vi "Configure Trigger.vi"(0 "VISA resource name":refnum<visa-resource-name>, 1 "Trigger Level (0.0 dBm)":dbl, 5 "Channel (1: Channel A)":u16(ring)=1 items=["Channel A"=1, "Channel B"=2], 7 "Trigger Source (3: Immediate)":u16(ring)=3 items=["Bus", "External", "Hold", "Immediate", "Internal A", "Internal B"], 9 "Trigger Slope (0: Positive)":u16(ring) items=["Positive", "Negative"], 11 "error in (no error)":errorcluster) -> (4 "VISA resource name out":refnum<visa-resource-name>, 15 "error out":errorcluster)   [LabVIEW 2020, in "Template - Power Meter.lvlib"]
doc: "Controls the behavior of the trigger system, including Trigger Source, Trigger Slope, and Trigger Level."
uses:
  <instrlib>/_Template - Power Meter/Template - Power Meter.lvlib
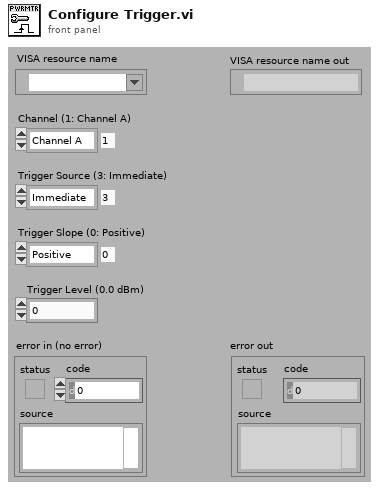
[diagram p1: front panel]
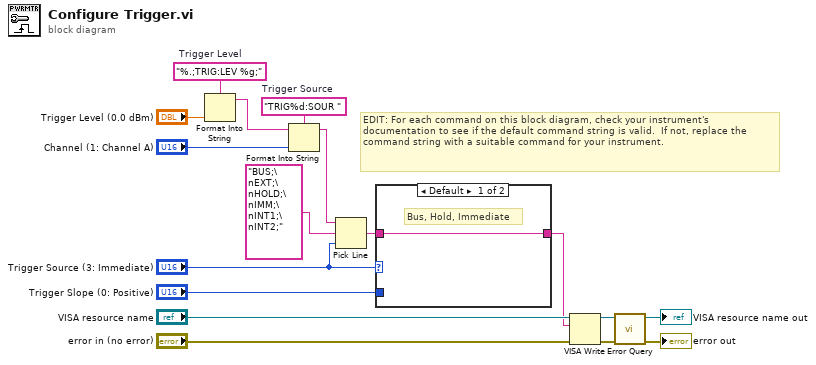
[diagram p0: block diagram]
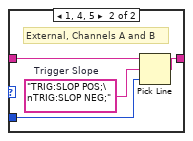
[diagram p2: hidden frame]
diagram:
  w10 = "TRIG%d:SOUR "  # Trigger Source
  w11 = "%.;TRIG:LEV %g;"  # Trigger Level
  # "EDIT: For each command on this block diagram, check your instrument's documentation to see if the default command string is valid.  If not, replace the command string with a suitable command for your instrument."
  n1 = Format Into String(format string=w11, "Trigger Level (0.0 dBm)") -> (resulting string=w6:string)  [unwired: 2 in, 1 out]
  n2 = Format Into String(format string=w10, initial string=w6, "Channel (1: Channel A)") -> (resulting string=w1:string)  [unwired: 1 in, 1 out]
  n3 = Pick Line(string ("")=w1, multi-line string="BUS;\nEXT;\nHOLD;\nIMM;\nINT1;\nINT2;", line index="Trigger Source (3: Immediate)") -> (output string=w2:string)
  n4 = case shown="Default" "Trigger Source (3: Immediate)" {
    tunnel: "Trigger Slope (0: Positive)" -> [_ w21]
    tunnel: [w18 w19] -> w3
    tunnel: w2 -> [w18 w20]
    frame Default {
      # "Bus, Hold, Immediate"
    }
    frame 1, 4, 5 {
      w22 = "TRIG:SLOP POS;\nTRIG:SLOP NEG;"  # Trigger Slope
      # "External, Channels A and B"
      n5 = Pick Line(string ("")=w20, multi-line string=w22, line index=w21) -> (output string=w19:string)
    }
  }
  n6 = VISA Write(VISA resource name="VISA resource name", write buffer=w3, error in (no error)="error in (no error)") -> (VISA resource name out=w15:refnum<visa-resource-name>, error out=w13:errorcluster)  [unwired: 1 out]
  n7 = call <instrlib>:"Error Query.vi"("error in (no error)"=w13, "VISA resource name"=w15) -> ("error out"=→"error out":errorcluster, "VISA resource name out"=→"VISA resource name out":refnum<visa-resource-name>)  [unwired: 6 in, 2 out]
